vi "Test_READ.vi"   [LabVIEW 2016]
doc: "Demonstrates how to initialize and write data to SD Card Shield. Once this example is executed successfully, you can run the SD Card - Read Data.vi shipping example to retrieve the data saved in the SD Card by this example and plot it on the screen of a host VI."
uses:
  <vilib>/Aledyne-TSXperts/Arduino Compatible Compiler for LabVIEW/Arduino Compatible Compiler for LabVIEW.lvlib
  <vilib>/Aledyne-TSXperts/Arduino Compatible Compiler for LabVIEW/Code Generator/Arduino APIs/Serial/Serial Settings.ctl
  <vilib>/Aledyne-TSXperts/Arduino Compatible Compiler for LabVIEW/Code Generator/Arduino APIs/SD Card/File Mode.ctl
panel:
  # "Overview: Demonstrates how to initialize and write data to SD Card Shield.  Once this example is executed successfully, you can run the SD Card - Read Data.vi shipping example to retrieve the data saved in the SD Card by this example and plot it on the screen of a host VI.\n\nInstructions:\n1. Stack the SD Card Shield on top of the Arduino board, as shown in the Figure below. \n2. Navigate to the block diagram and look at the data being written to the SD Card. Feel free to modify the two constants that get written to the SD Card to see the effect of the changes.\n3. Open and run the shipping example project SD Card - Read Data and run the host VI. Note how the constant data written to the SD Card on this VI is displayed in the SD Card - Data Read - Host.vi."
types:
  T1 = typedef "Arduino Compatible Compiler for LabVIEW.lvlib/File Mode.ctl" = enum16{"Read", "Write_Read"}
  T2 = typedef "Arduino Compatible Compiler for LabVIEW.lvlib/Serial Settings.ctl" = u16
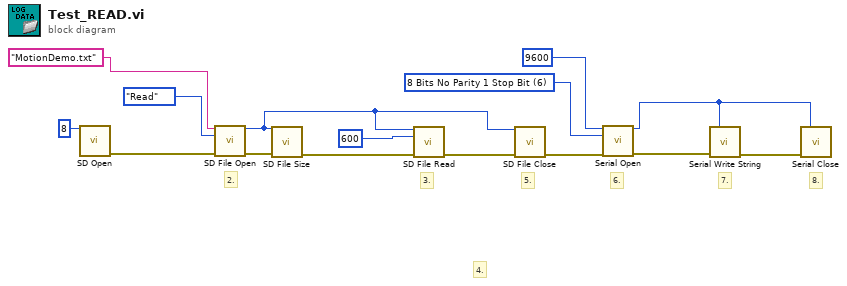
[diagram p0: block diagram]
diagram:
  w14 = T2 6 items=["5 Bits No Parity 1 Stop Bit"=0, "6 Bits No Parity 1 Stop Bit"=2, "7 Bits No Parity 1 Stop Bit"=4, "8 Bits No Parity 1 Stop Bit"=6, "5 Bits No Parity 2 Stop Bits"=8, "6 Bits No Parity 2 Stop Bits"=10, "7 Bits No Parity 2 Stop Bits"=12, "8 Bits No Parity 2 Stop Bits"=14, "5 Bits Even Parity 1 Stop Bits"=32, "6 Bits Even Parity 1 Stop Bits"=34, "7 Bits Even Parity 1 Stop Bits"=36, "8 Bits Even Parity 1 Stop Bits"=38, "5 Bits Even Parity 2 Stop Bits"=40, "6 Bits Even Parity 2 Stop Bits"=42, "7 Bits Even Parity 2 Stop Bits"=44, "8 Bits Even Parity 2 Stop Bits"=46, "5 Bits Odd Parity 1 Stop Bits"=48, "6 Bits Odd Parity 1 Stop Bits"=50, "7 Bits Odd Parity 1 Stop Bits"=52, "8 Bits Odd Parity 1 Stop Bits"=54, "5 Bits Odd Parity 2 Stop Bits"=56, "6 Bits Odd Parity 2 Stop Bits"=58, "7 Bits Odd Parity 2 Stop Bits"=60, "8 Bits Odd Parity 2 Stop Bits"=62] ("Serial Settings")
  # "7."
  # "6."
  # "5."
  # "4."
  # "8."
  # "3."
  # "2."
  n1 = call <vilib>:"SD Open.vi"("CS Pin"=u8 8) -> ("error out"=w7:errorcluster)  [unwired: 13 in, 1 out]
  n2 = call <vilib>:"SD File Open.vi"("File"="MotionDemo.txt" ("Directory"), "Mode"=File_Mode."Read", "error in (no error)"=w7) -> ("File Reference"=w5:i32, "error out"=w3:errorcluster)  [unwired: 10 in, 1 out]
  n3 = call <vilib>:"SD File Size.vi"("Reference"=w5, "error in (no error)"=w3) -> ("bytes"=w1:u32, "error out"=w4:errorcluster)  [unwired: 12 in]
  n4 = call <vilib>:"SD File Read.vi"("Reference"=w5, "Length"=600, "error in (no error)"=w4) -> ("error out"=w12:errorcluster)  [unwired: 11 in, 1 out]
  n5 = call <vilib>:"SD File Close.vi"("Reference"=w5, "error in (no error)"=w12) -> ("error out"=w11:errorcluster)  [unwired: 13 in]
  n6 = call <vilib>:"Serial Open.vi"("Speed"=u32 9600, "Serial Settings"=w14, "error in (no error)"=w11) -> ("Instance"=w9:u8, "error out"=w8:errorcluster)  [unwired: 11 in]
  n7 = call <vilib>:"Serial Write String.vi"("Instance"=w9, "error in (no error)"=w8) -> ("error out"=w10:errorcluster)  [unwired: 13 in]
  n8 = call <vilib>:"Serial Close.vi"("Instance"=w9, "error in (no error)"=w10) -> ()  [unwired: 13 in, 1 out]
